vi "laneleftright41.vi"() -> (2 "Coeff right":dbl[](array[numeric]), 3 "Coeff left":dbl[](array[numeric]))   [LabVIEW 2015]
uses:
  G_SEN.vi
  <vilib>/Analysis/1siggen.llb/Ramp Pattern by Delta.vi
  G_LCM.vi
  <vilib>/Analysis/polynomials.llb/1D Polynomial Evaluation (DBL).vi
  G_ALL.vi
  <vilib>/Analysis/NI_AALPro.lvlib
  <vilib>/Analysis/NI_AALBase.lvlib
panel:
  out "y 2":dbl[](array[numeric])
  out "x 2":dbl[](array[numeric])
  out "w 2":dbl[](array[numeric])
  out "lane_right_pt":dbl[][](array[numeric])
  in  "x_gain":dbl=1.0 min=-1.0 max=1.0
  in  "y_gain":dbl=1.0 min=-1.0 max=1.0
  out "map_track 2":dbl[][](array[numeric])
  in  "d_safe":dbl=1.1 format="%#_13g"
  out "map_track":dbl[][](array[numeric])
  out "lane_left_pt":dbl[][](array[numeric])
  out "x_shift":dbl format="%#_13g"
  out "y_shift":dbl format="%#_13g"
  in  "lane_gain":dbl=0.7 min=-1.0 max=1.0
  out "Lane_C_M":dbl[](array[numeric])=[0.8601491478953653, 0.8717844136967624, 0.882947592858927, 0.8936326403234123, 0.9038337699485205, 0.9135454576426009, 0.9227624443554423, 0.9314797389261423, 0.9396926207859084, 0.9473966425143293, 0.9545876322477319, 0.9612616959383189, 0.9674152194628639, 0.9730448705798238, 0.9781476007338057, 0.9827206467064133, 0.9867615321125792, 0.9902680687415704, 0.993238357741943, 0.9956707906498045, 0.9975640502598242, 0.9989171113385246, 0.9997292411794617, 1.0, 0.9997292411794617, 0.9989171113385246, 0.9975640502598242, 0.9956707906498045, 0.993238357741943, 0.9902680687415704, 0.9867615321125792, 0.9827206467064133]
  out "ratio(-1:left1:right)":dbl
  out "NaN/Path/Refnum?":bool
  out "Rleft":dbl
  out "Rright":dbl
  in  "poly":i32=2 min=1 max=5 step=1
  out "Coeff stop":dbl[](array[numeric])
  out "y_end":dbl[](array[numeric])=[0.8601491478953653, 0.8717844136967624, 0.882947592858927, 0.8936326403234123, 0.9038337699485205, 0.9135454576426009, 0.9227624443554423, 0.9314797389261423, 0.9396926207859084, 0.9473966425143293, 0.9545876322477319, 0.9612616959383189, 0.9674152194628639, 0.9730448705798238, 0.9781476007338057, 0.9827206467064133, 0.9867615321125792, 0.9902680687415704, 0.993238357741943, 0.9956707906498045, 0.9975640502598242, 0.9989171113385246, 0.9997292411794617, 1.0, 0.9997292411794617, 0.9989171113385246, 0.9975640502598242, 0.9956707906498045, 0.993238357741943, 0.9902680687415704, 0.9867615321125792, 0.9827206467064133]
  in  "iter":i32=7
  out "Waveform Graph":dbl[](graph)
  out "w":dbl[](array[numeric])
  out "XY Graph 4":cluster{"Y":dbl[], "Y":dbl[]}[](graph)=[{"Y"=array[3210 elements], "Y"=array[3210 elements]}, {"Y"=[-0.0, 0.001154394197769193, 0.004617650635850623, 0.010389990872226917, 0.018471784248973222, 0.02886354801042046, 0.041565947468740205, 0.056579796217107514, 0.0739060563904701, 0.0935458389742223, 0.11550040416098284, 0.13977116175580306, 0.16635967162997645, 0.19526764422393228, 0.2264969410994837, 0.26004957554195585, 0.2959277132125635, 0.3341336728515216, 0.374669927032528, 0.417539102969144, 0.4627439833735707, 0.5102875073687159, 0.560172771454063, 0.6124030305261954, 0.6669816989546717, 0.7239123517142048, 0.7831987255740245, 0.8448447203451934, 0.9088544001870815, 0.975231994973953, 1.0439819017227023, 1.1151086860829622, 1.1886170838907617, 1.2645120027869723, 1.342798523901962, 1.42348190360768, 1.5065675753387922, 1.592061151484188, 1.6799684253507792, 1.770295373200753, 1.8630481563645134, 1.9582331234307588, 2.0558568125157564, 2.1559259536137603, 2.258447471030621], "Y"=[0.0, 0.5, 1.0, 1.5, 2.0, 2.5, 3.0, 3.5, 4.0, 4.5, 5.0, 5.5, 6.0, 6.5, 7.0, 7.5, 8.0, 8.5, 9.0, 9.5, 10.0, 10.5, 11.0, 11.5, 12.0, 12.5, 13.0, 13.5, 14.0, 14.5, 15.0, 15.5, 16.0, 16.5, 17.0, 17.5, 18.0, 18.5, 19.0, 19.5, 20.0, 20.5, 21.0, 21.5, 22.0]}, {"Y"=[0.362252581831572], "Y"=[-0.8199241909738847]}, {"Y"=array[210 elements], "Y"=array[210 elements]}, {"Y"=[-0.925, -0.925, -0.925, -0.6775, -0.6775, -0.925, -0.925, -0.925, -0.925, -0.6775, -0.6775, -0.925, -0.925, -0.925, 0.9025, 0.9025, 0.9025, 0.6775, 0.6775, 0.9025, 0.9025, 0.9025, 0.9025, 0.6775, 0.6775, 0.9025, 0.9025, 0.9025, -0.925], "Y"=[-0.75, -0.224, 0.224, 0.224, -0.224, -0.224, 0.224, 2.415, 2.885, 2.885, 2.415, 2.415, 2.885, 3.5, 3.5, 2.885, 2.415, 2.415, 2.885, 2.885, 2.415, 0.224, -0.224, -0.224, 0.224, 0.224, -0.224, -0.75, -0.75]}, {"Y"=[0.171875, 0.15377271904051304, 0.1346290179491043, 0.11445423440635205, 0.09325870609283447, 0.07105277068912982, 0.04784676587581635, 0.02365102933347224, -0.0015241012573242174, -0.02766828821599482, -0.05477119386196136, -0.08282248051464558, -0.11181181049346922, -0.14172884611785413, -0.17256324970722198, -0.20430468358099463, -0.23694281005859374, -0.27046729145944115, -0.30486779010295867, -0.340133968308568, -0.3762554883956909, -0.41322201268374914, -0.4510232034921646, -0.4896487231403589], "Y"=[0.0, 0.5, 1.0, 1.5, 2.0, 2.5, 3.0, 3.5, 4.0, 4.5, 5.0, 5.5, 6.0, 6.5, 7.0, 7.5, 8.0, 8.5, 9.0, 9.5, 10.0, 10.5, 11.0, 11.5]}, {"Y"=[1.796875, 1.778772719040513, 1.7596290179491043, 1.739454234406352, 1.7182587060928345, 1.6960527706891297, 1.6728467658758164, 1.6486510293334722, 1.6234758987426758, 1.5973317117840051, 1.5702288061380387, 1.5421775194853544, 1.513188189506531, 1.483271153882146, 1.452436750292778, 1.4206953164190055, 1.3880571899414063, 1.354532708540559, 1.3201322098970414, 1.284866031691432, 1.248744511604309, 1.2117779873162509, 1.1739767965078354, 1.135351276859641, 1.0959117660522462, 1.0556686017662287, 1.014632121682167, 0.9728126634806396, 0.9302205648422242, 0.8868661634474992], "Y"=[0.0, 0.5, 1.0, 1.5, 2.0, 2.5, 3.0, 3.5, 4.0, 4.5, 5.0, 5.5, 6.0, 6.5, 7.0, 7.5, 8.0, 8.5, 9.0, 9.5, 10.0, 10.5, 11.0, 11.5, 12.0, 12.5, 13.0, 13.5, 14.0, 14.5]}, {"Y"=[-1.453125, -1.471227280959487, -1.4903709820508957, -1.510545765593648, -1.5317412939071655, -1.5539472293108703, -1.5771532341241836, -1.6013489706665278, -1.6265241012573242, -1.6526682882159949, -1.6797711938619613, -1.7078224805146456, -1.736811810493469, -1.766728846117854, -1.797563249707222, -1.8293046835809945, -1.8619428100585937, -1.895467291459441, -1.9298677901029586], "Y"=[0.0, 0.5, 1.0, 1.5, 2.0, 2.5, 3.0, 3.5, 4.0, 4.5, 5.0, 5.5, 6.0, 6.5, 7.0, 7.5, 8.0, 8.5, 9.0]}, {"Y"=[0.171875, 0.2568230007600336, 0.3384052130063493, 0.44574342526006827, 0.5205081969556753, 0.5917680690742042, 0.659409530134929, 0.7229937549325056, 0.7835496148685115, 0.8405449546633443, 0.9258576868463875], "Y"=[-20.239964538708662, -19.725637940364884, -19.211158961966362, -18.6998967366845, -18.19022720070031, -17.681887266143153, -17.17615515566314, -16.67683575591291, -16.176265245349786, -15.679082775270938, -15.183754484614711]}, {"Y"=[7.134647485270904], "Y"=[38.71960961082238]}, {"Y"=array[980 elements], "Y"=array[980 elements]}, {"Y"=[], "Y"=[]}]
  out "y":dbl[](array[numeric])
  out "x":dbl[](array[numeric])
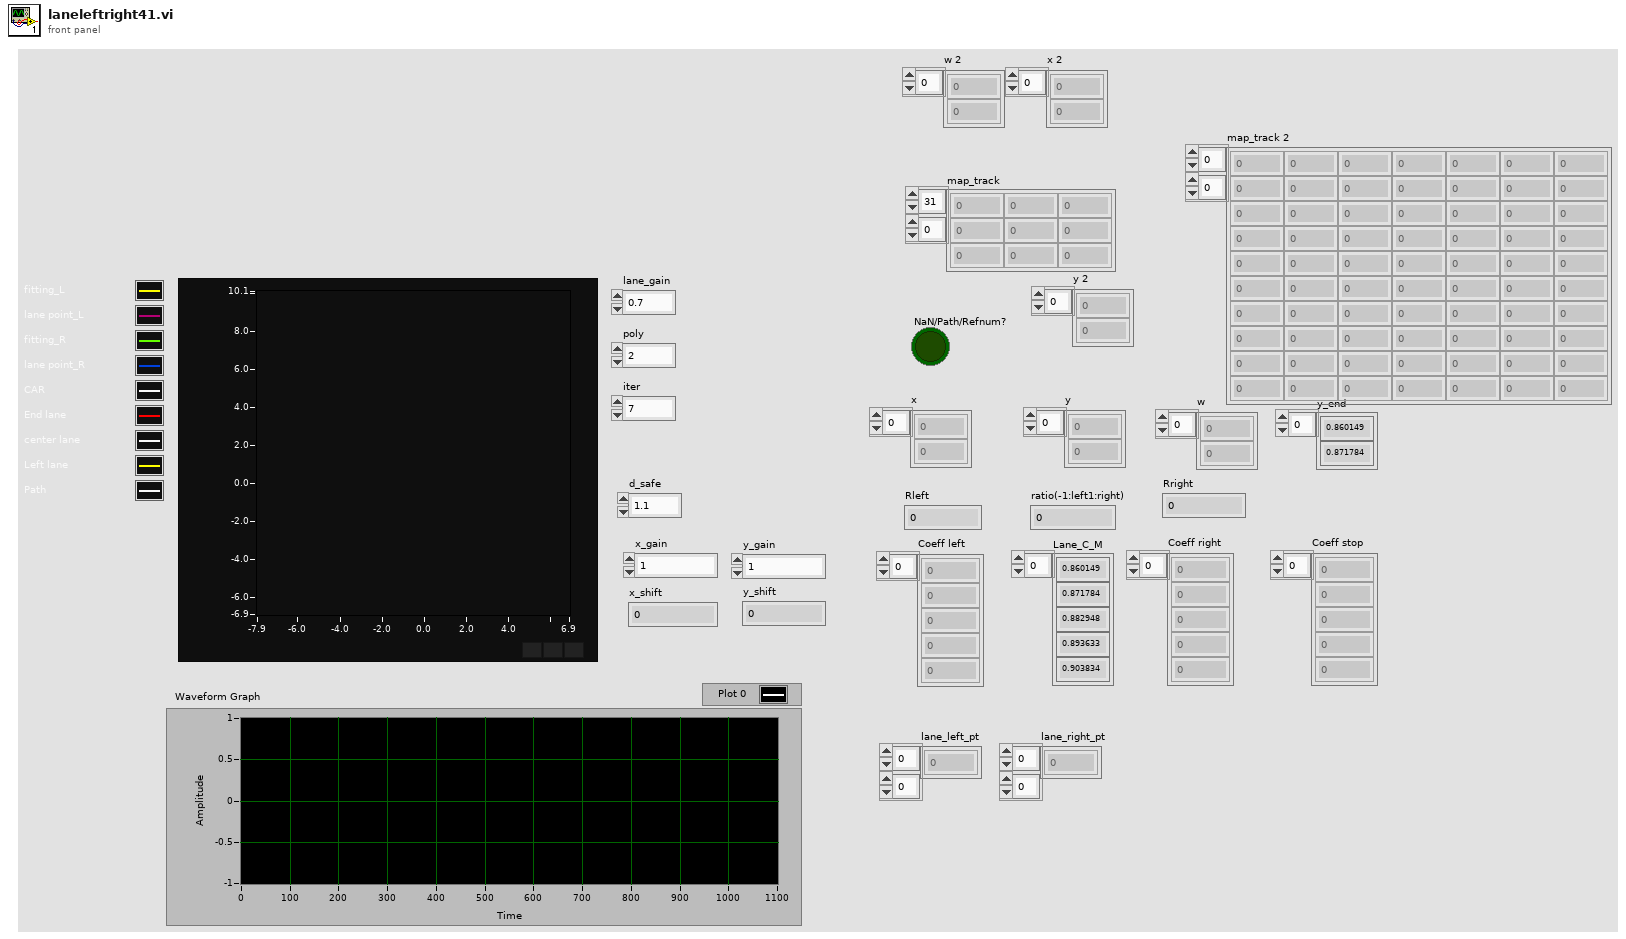
[diagram p1: front panel]
types:
  T1 = cluster{"hash":i64, "sys time":i64, "size":i64, "x":dbl[], "y":dbl[]}
  T2 = cluster{"delta":bool, "Rotational position":dbl, "Rotational position":dbl}[]
  T3 = cluster{"C_Wheel base":dbl, "ratio_steer":dbl, "Overall width":dbl, "af":dbl, "turn radius":dbl, "eval":dbl, "ap":dbl, "an":dbl, "Vmax":dbl, "mu":dbl, "Vlast":dbl}
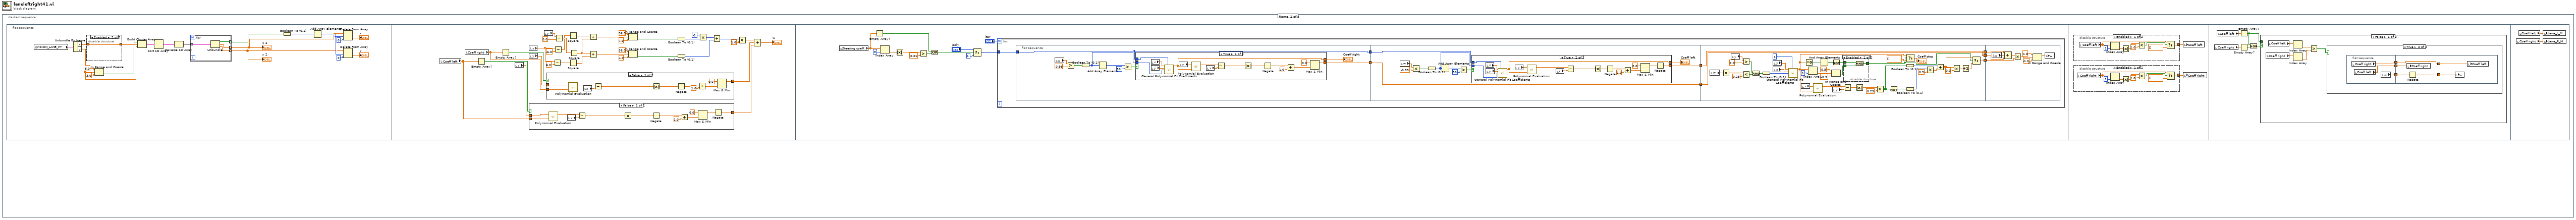
[diagram p0: block diagram]
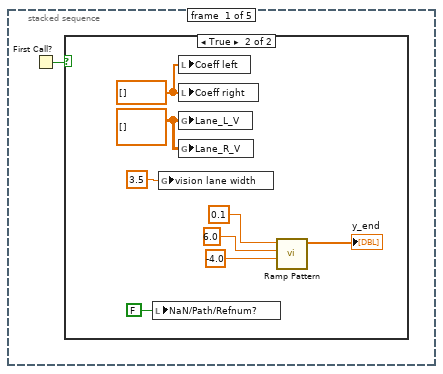
[diagram p2: hidden frame]
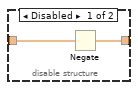
[diagram p4: hidden frame]
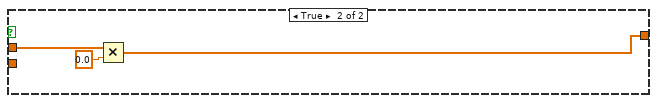
[diagram p5: hidden frame]
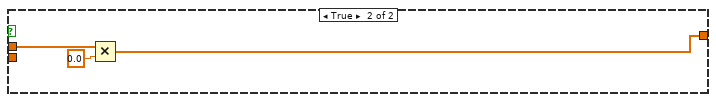
[diagram p6: hidden frame]
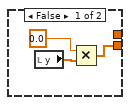
[diagram p7: hidden frame]
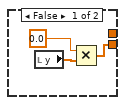
[diagram p8: hidden frame]
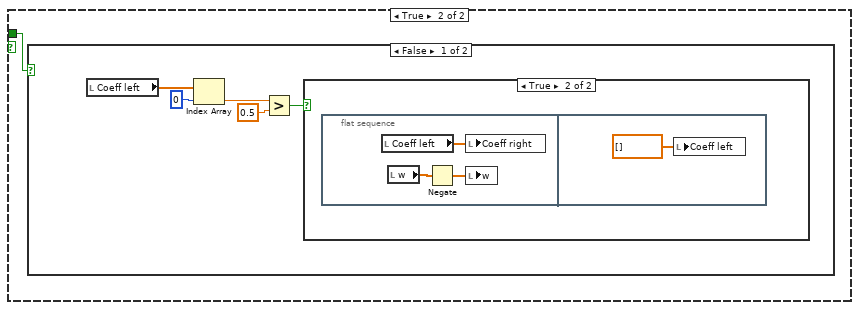
[diagram p13: hidden frame]
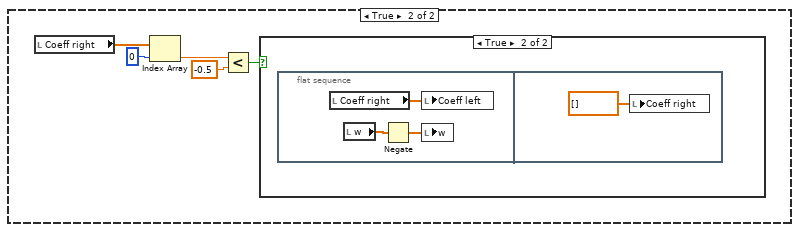
[diagram p15: hidden frame]
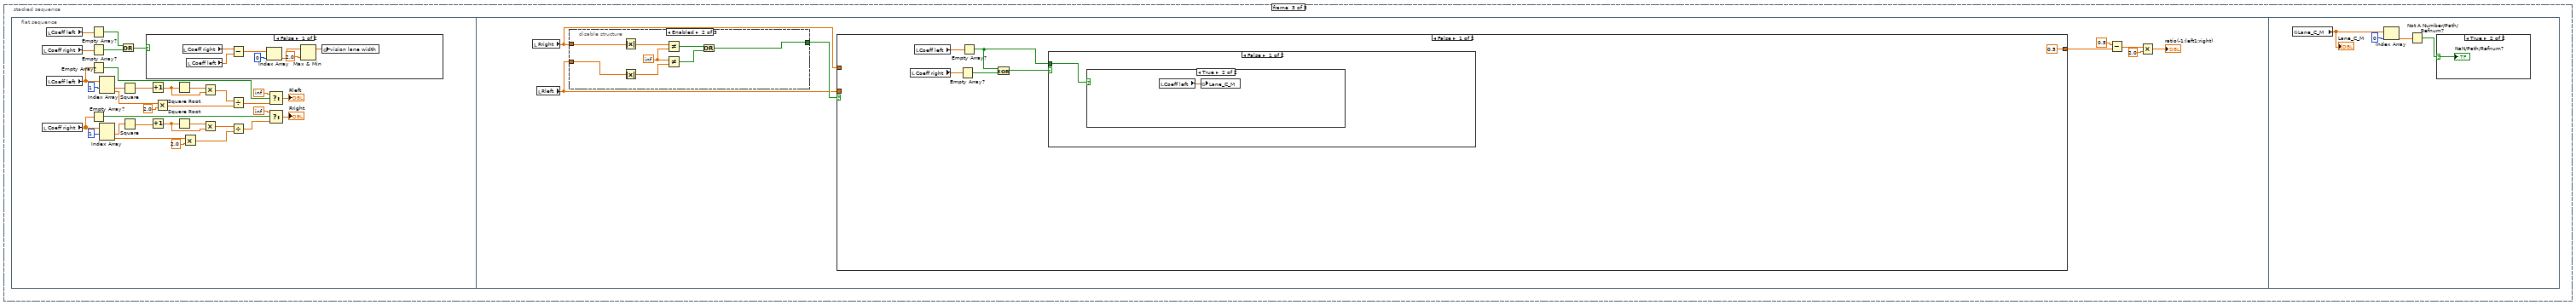
[diagram p17: hidden frame]
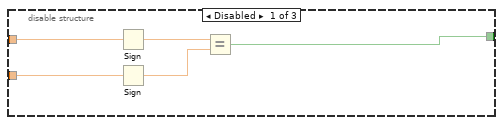
[diagram p19: hidden frame]
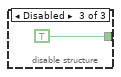
[diagram p20: hidden frame]
diagram:
  n1 = stacked-sequence {
    frame #0 {
      n2 = First Call?() -> (First Call?: T/F=w1:bool)
      n3 = case shown="True" w1 {
        frame False {
        }
        frame True {
          w2 = dbl[] [] ("Coeff left")
          w4 = dbl[][] [] ("Lane_R_V")
          n4 = local write "NaN/Path/Refnum?"(FALSE ("NaN/Path/Refnum?")) -> ()
          n5 = global write "G_SEN.vi" "vision lane width"(3.5 ("vision lane width")) -> ()
          n6 = local write "Coeff left"(w2) -> ()
          n7 = local write "Coeff right"(w2) -> ()
          n8 = global write "G_SEN.vi" "Lane_L_V"(w4) -> ()
          n9 = global write "G_SEN.vi" "Lane_R_V"(w4) -> ()
          n10 = call-poly <vilib>:"Ramp Pattern.vi"("start"=-4.0, "end"=6.0, "delta"=0.1) -> ("Ramp Pattern"=→"y_end":dbl[])  [unwired: 6 in, 2 out]
        }
      }
    }
    frame #1 {
      n11 = flat-sequence {
        frame #0 {
          n12 = global read "G_LCM.vi" "VISION_LANE_PT"() -> (w12:T1)
          n13 = Unbundle By Name(w12) -> ("x"=w27:dbl[], "y"=w21:dbl[])
          n14 = disable-structure shown="Enabled" {
            disable-tunnel: w27 -> [w30 w31]
            disable-tunnel: [w29 w31] -> w28
            frame Disabled {
              n15 = Negate(x=w30) -> (-x=w29:dbl[])
            }
            frame Enabled {
            }
          }
          n16 = In Range and Coerce(upper limit=8.0 ("delta"), x=w21, lower limit=-3.0) -> (In Range?=w19:bool[])  [unwired: 1 out]
          n17 = Build Cluster Array(w19, w28, w21) -> (w17:T2)
          n18 = Sort 1D Array(array=w17) -> (sorted array=w18:T2)
          n19 = Reverse 1D Array(array=w18) -> (reversed array=w14:T2)
          n20 = for {
            tunnel: w14 -> [w35] mode=indexing
            tunnel: [w34] -> w11 mode=indexing
            tunnel: [w33] -> w10 mode=indexing
            tunnel: [w32] -> w22 mode=indexing
            n21 = Unbundle(w35) -> ("delta"=w32:bool, "Rotational position"=w34:dbl, "Rotational position"=w33:dbl)
          }
          "x 2" <- w11
          "y 2" <- w10
          n22 = Boolean To (0,1)(Boolean=w22) -> (0, 1=w15:i16[])
          n23 = Add Array Elements(numeric array=w15) -> (sum=w23:i16)
          n24 = Delete From Array(array=w11, length=w23, index=0) -> (deleted portion=→"x":dbl[])  [unwired: 1 out]
          n25 = Delete From Array(array=w10, length=w23, index=0) -> (deleted portion=→"y":dbl[])  [unwired: 1 out]
        }
        frame #1 {
          n26 = local read "Coeff left"() -> (w67:dbl[])
          n27 = local read "Coeff right"() -> (w66:dbl[])
          n28 = Empty Array?(array=w67) -> (empty?=w68:bool)
          n29 = Empty Array?(array=w66) -> (empty?=w69:bool)
          n30 = local read "y"() -> (w64:dbl[])
          n31 = local read "x"() -> (w36:dbl[])
          n32 = local read "y"() -> (w70:dbl[])
          n33 = case shown="False" w68 {
            tunnel: w64 -> [w90 w98]
            tunnel: w67 -> [w87 _]
            tunnel: [w85 w97] -> w65
            frame False {
              n34 = call-poly <vilib>:"Polynomial Evaluation.vi"("P(x)"=w87, "A"=w90) -> ("P(A)"=w89:dbl[])  [unwired: 1 out]
              n35 = local read "x"() -> (w88:dbl[])
              n36 = Subtract(x=w89, y=w88) -> (x-y=w94:dbl[])
              n37 = Absolute Value(x=w94) -> (abs(x)=w93:dbl[])
              n38 = Negate(x=w93) -> (-x=w92:dbl[])
              n39 = Add(x=w92, y=1.0) -> (x+y=w96:dbl[])
              n40 = Max & Min(x=0.0, y=w96) -> (max(x,y)=w86:dbl[])  [unwired: 1 out]
              n41 = Negate(x=w86) -> (-x=w85:dbl[])
            }
            frame True {
              n42 = Multiply(x=w98, y=0.0) -> (x*y=w97:dbl[])
            }
          }
          n43 = local read "y"() -> (w37:dbl[])
          n44 = case shown="False" w69 {
            tunnel: [w79 w82] -> w62
            tunnel: w66 -> [w78 _]
            tunnel: w70 -> [w71 w83]
            frame False {
              n45 = call-poly <vilib>:"Polynomial Evaluation.vi"("P(x)"=w78, "A"=w71) -> ("P(A)"=w76:dbl[])  [unwired: 1 out]
              n46 = local read "x"() -> (w77:dbl[])
              n47 = Subtract(x=w76, y=w77) -> (x-y=w72:dbl[])
              n48 = Absolute Value(x=w72) -> (abs(x)=w73:dbl[])
              n49 = Negate(x=w73) -> (-x=w74:dbl[])
              n50 = Add(x=w74, y=1.0) -> (x+y=w80:dbl[])
              n51 = Max & Min(x=0.0, y=w80) -> (max(x,y)=w79:dbl[])  [unwired: 1 out]
            }
            frame True {
              n52 = Multiply(x=w83, y=0.0) -> (x*y=w82:dbl[])
            }
          }
          n53 = Subtract(x=w36, y=6.0) -> (x-y=w40:dbl[])
          n54 = Subtract(x=w36, y=-6.0) -> (x-y=w42:dbl[])
          n55 = Subtract(x=w37, y=0.0) -> (x-y=w49:dbl[])
          n56 = Square(x=w42) -> (x^2=w41:dbl[])
          n57 = Square(x=w40) -> (x^2=w50:dbl[])
          n58 = Square(x=w49) -> (x^2=w51:dbl[])
          n59 = Add(x=w41, y=w51) -> (x+y=w57:dbl[])
          n60 = Add(x=w51, y=w50) -> (x+y=w52:dbl[])
          n61 = In Range and Coerce(upper limit=36.0, x=w57, lower limit=4.0) -> (In Range?=w59:bool[])  [unwired: 1 out]
          n62 = In Range and Coerce(upper limit=36.0, x=w52, lower limit=4.0) -> (In Range?=w58:bool[])  [unwired: 1 out]
          n63 = Boolean To (0,1)(Boolean=w59) -> (0, 1=w60:i16[])
          n64 = Boolean To (0,1)(Boolean=w58) -> (0, 1=w61:i16[])
          n65 = Multiply(x=i16 -1, y=w60) -> (x*y=w45:i16[])
          n66 = Add(x=w45, y=w61) -> (x+y=w47:i16[])
          n67 = Multiply(x=w47, y=1.0 ("element")) -> (x*y=w63:dbl[])
          n68 = Compound Arithmetic op=ADD(w63, w62, w65) -> (→"w":dbl[])
        }
        frame #2 {
          n69 = global read "G_ALL.vi" "Steering coeff"() -> (w107:dbl[])
          n70 = Empty Array?(array=w107) -> (empty?=w110:bool)
          n71 = Index Array(array=w107, index=3) -> (element=w105:dbl)
          n72 = Absolute Value(x=w105) -> (abs(x)=w104:dbl)
          n73 = Greater?(x=w104, y=0.01) -> (0:w102:bool)
          n74 = Or(x=w110, y=w102) -> (x .or. y?=w109:bool)
          n75 = Select(t="poly", s=w109, f=1) -> (s? t:f=w100:i32)
          n76 = for {
            N: "iter" -> [_]
            tunnel: w100 -> [w113]
            n77 = flat-sequence {
              tunnel: [w127] -> w119
              tunnel: w113 -> [w120]
              tunnel: [w120] -> w112
              tunnel: [w158] -> w118
              tunnel: w119 -> [w158]
              tunnel: [w155] -> w116
              tunnel: w112 -> [w148]
              tunnel: w118 -> [w220]
              tunnel: [w220] -> w117
              tunnel: w116 -> [w219]
              tunnel: [w219] -> w115
              tunnel: [w190] -> w114
              tunnel: w117 -> [w228]
              tunnel: w115 -> [w224]
              tunnel: w114 -> [w226]
              frame #0 {
                n78 = local read "w"() -> (w129:dbl[])
                n79 = Greater?(x=w129, y=0.99) -> (0:w121:bool[])
                n80 = Boolean To (0,1)(Boolean=w121) -> (0, 1=w122:i16[])
                n81 = Add Array Elements(numeric array=w122) -> (sum=w125:i16)
                n82 = Greater?(x=w125, y=i16 50) -> (0:w123:bool)
                n83 = case shown="True" w123 {
                  tunnel: [w131 w138] -> w127
                  tunnel: [_ w137] -> w126
                  tunnel: w122 -> [_ w134]
                  tunnel: w120 -> [_ w133]
                  frame False {
                    n84 = local read "y"() -> (w132:dbl[])
                    n85 = Multiply(x=0.0, y=w132) -> (x*y=w131:dbl[])
                  }
                  frame True {
                    n86 = local read "x"() -> (w135:dbl[])
                    n87 = local read "y"() -> (w136:dbl[])
                    n88 = call <vilib>:"General Polynomial Fit Coefficients.vi"("Y"=w135, "polynomial order"=w133, "X"=w136, "Weight"=w134) -> ("Polynomial Coefficients"=w137:dbl[])  [unwired: 10 in, 1 out]
                    n89 = local read "y"() -> (w147:dbl[])
                    n90 = call-poly <vilib>:"Polynomial Evaluation.vi"("P(x)"=w137, "A"=w147) -> ("P(A)"=w146:dbl[])  [unwired: 1 out]
                    n91 = local read "x"() -> (w145:dbl[])
                    n92 = Subtract(x=w146, y=w145) -> (x-y=w144:dbl[])
                    n93 = Absolute Value(x=w144) -> (abs(x)=w143:dbl[])
                    n94 = Negate(x=w143) -> (-x=w142:dbl[])
                    n95 = Add(x=w142, y=1.0) -> (x+y=w139:dbl[])
                    n96 = Max & Min(x=0.0, y=w139) -> (max(x,y)=w138:dbl[])  [unwired: 1 out]
                  }
                }
                "Coeff right" <- w126
              }
              frame #1 {
                n97 = local read "w"() -> (w156:dbl[])
                n98 = Less?(x=w156, y=-0.99) -> (x < y?=w151:bool[])
                n99 = Boolean To (0,1)(Boolean=w151) -> (0, 1=w149:i16[])
                n100 = Add Array Elements(numeric array=w149) -> (sum=w152:i16)
                n101 = Greater?(x=w152, y=i16 50) -> (0:w150:bool)
                n102 = case shown="True" w150 {
                  tunnel: [w159 w167] -> w155
                  tunnel: [_ w166] -> w154
                  tunnel: w149 -> [_ w163]
                  tunnel: w148 -> [_ w162]
                  frame False {
                    n103 = local read "y"() -> (w160:dbl[])
                    n104 = Multiply(x=0.0, y=w160) -> (x*y=w159:dbl[])
                  }
                  frame True {
                    n105 = local read "x"() -> (w164:dbl[])
                    n106 = local read "y"() -> (w165:dbl[])
                    n107 = call <vilib>:"General Polynomial Fit Coefficients.vi"("Y"=w164, "polynomial order"=w162, "X"=w165, "Weight"=w163) -> ("Polynomial Coefficients"=w166:dbl[])  [unwired: 10 in, 1 out]
                    n108 = local read "y"() -> (w171:dbl[])
                    n109 = call-poly <vilib>:"Polynomial Evaluation.vi"("P(x)"=w166, "A"=w171) -> ("P(A)"=w172:dbl[])  [unwired: 1 out]
                    n110 = local read "x"() -> (w173:dbl[])
                    n111 = Subtract(x=w172, y=w173) -> (x-y=w174:dbl[])
                    n112 = Absolute Value(x=w174) -> (abs(x)=w175:dbl[])
                    n113 = Negate(x=w175) -> (-x=w169:dbl[])
                    n114 = Add(x=w169, y=1.0) -> (x+y=w176:dbl[])
                    n115 = Max & Min(x=0.0, y=w176) -> (max(x,y)=w170:dbl[])  [unwired: 1 out]
                    n116 = Negate(x=w170) -> (-x=w167:dbl[])
                  }
                }
                "Coeff left" <- w154
              }
              frame #2 {
                n117 = local read "w"() -> (w198:dbl[])
                n118 = Absolute Value(x=w198) -> (abs(x)=w197:dbl[])
                n119 = local read "y"() -> (w202:dbl[])
                n120 = Greater?(x=w202, y=2.0) -> (0:w200:bool[])
                n121 = Less?(x=w197, y=0.25) -> (x < y?=w196:bool[])
                n122 = And(x=w200, y=w196) -> (x .and. y?=w199:bool[])
                n123 = Boolean To (0,1)(Boolean=w199) -> (0, 1=w218:i16[])
                n124 = local read "y"() -> (w212:dbl[])
                n125 = local read "x"() -> (w211:dbl[])
                n126 = call <vilib>:"General Polynomial Fit Coefficients.vi"("Y"=w212, "polynomial order"=1, "X"=w211, "Weight"=w218) -> ("Polynomial Coefficients"=w183:dbl[])  [unwired: 10 in, 1 out]
                n127 = local read "x"() -> (w216:dbl[])
                n128 = Equal To 0?(x=w183) -> (x = 0?=w182:bool[])
                n129 = Index Array(array=w183, index=1) -> (element=w193:dbl)
                n130 = call-poly <vilib>:"Polynomial Evaluation.vi"("P(x)"=w183, "A"=w216) -> ("P(A)"=w215:dbl[])  [unwired: 1 out]
                n131 = And Array Elements(Boolean array=w182) -> (logical AND=w179:bool)
                n132 = In Range and Coerce(upper limit=0.5, x=w193, lower limit=-0.5) -> (In Range?=w181:bool)  [unwired: 1 out]
                n133 = Not(x=w179) -> (.not. x?=w178:bool)
                n134 = local read "y"() -> (w214:dbl[])
                n135 = Subtract(x=w215, y=w214) -> (x-y=w213:dbl[])
                n136 = disable-structure shown="Enabled" {
                  disable-tunnel: w181 -> [w223 _]
                  disable-tunnel: [w222 _] -> w180
                  disable-tunnel: w178 -> [w221 _]
                  frame Enabled {
                    n137 = And(x=w221, y=w223) -> (x .and. y?=w222:bool)
                  }
                  frame Disabled {
                  }
                }
                n138 = Absolute Value(x=w213) -> (abs(x)=w210:dbl[])
                n139 = Greater?(x=w210, y=0.25 ("Numeric 2")) -> (0:w208:bool[])
                n140 = Not(x=w208) -> (.not. x?=w207:bool[])
                n141 = Boolean To (0,1)(Boolean=w208) -> (0, 1=w203:i16[])
                n142 = Boolean To (0,1)(Boolean=w207) -> (0, 1=w206:i16[])
                n143 = Select(t=w183, s=w180, f=dbl[] []) -> (s? t:f=→"Coeff stop":dbl[])
                n144 = Multiply(x=w206, y=0.5) -> (x*y=w204:dbl[])
                n145 = Add(x=w203, y=w204) -> (x+y=w189:dbl[])
                n146 = Multiply(x=w189, y=0.0) -> (x*y=w187:dbl[])
                n147 = Increment(x=w187) -> (x+1=w186:dbl[])
                n148 = Select(t=w189, s=w180, f=w186) -> (s? t:f=w190:dbl[])
              }
              frame #3 {
                n149 = local read "w"() -> (w232:dbl[])
                n150 = Compound Arithmetic op=ADD(w224, w232, w228) -> (w225:dbl[])
                n151 = Multiply(x=w225, y=w226) -> (x*y=w227:dbl[])
                n152 = In Range and Coerce(upper limit=1.0, x=w227, lower limit=-1.0) -> (coerced(x)=w229:dbl[])  [unwired: 1 out]
                n153 = local write "w"(w229) -> ()
              }
            }
          }
        }
        frame #3 {
          n154 = disable-structure shown="Enabled" {
            disable-tunnel: [w236 _] -> w233
            frame Enabled {
              n155 = local read "Coeff left"() -> (w235:dbl[])
              n156 = Index Array(array=w235, index=1) -> (element=w238:dbl)
              n157 = Absolute Value(x=w238) -> (abs(x)=w239:dbl)
              n158 = Less?(x=w239, y=1.0) -> (x < y?=w241:bool)
              n159 = Select(t=w235, s=w241, f=dbl[] []) -> (s? t:f=w236:dbl[])
            }
            frame Disabled {
            }
          }
          n160 = disable-structure shown="Enabled" {
            disable-tunnel: [w245 _] -> w234
            frame Enabled {
              n161 = local read "Coeff right"() -> (w243:dbl[])
              n162 = Index Array(array=w243, index=1) -> (element=w249:dbl)
              n163 = Absolute Value(x=w249) -> (abs(x)=w248:dbl)
              n164 = Less?(x=w248, y=1.0) -> (x < y?=w246:bool)
              n165 = Select(t=w243, s=w246, f=dbl[] []) -> (s? t:f=w245:dbl[])
            }
            frame Disabled {
            }
          }
          n166 = local write "Coeff left"(w233) -> ()
          n167 = local write "Coeff right"(w234) -> ()
        }
        frame #4 {
          n168 = local read "Coeff right"() -> (w252:dbl[])
          n169 = local read "Coeff left"() -> (w251:dbl[])
          n170 = Empty Array?(array=w251) -> (empty?=w255:bool)
          n171 = Empty Array?(array=w252) -> (empty?=w253:bool)
          n172 = Exclusive Or(1:w253, 2:w255) -> (0:w254:bool)
          n173 = case shown="False" w254 {
            tunnel: w255 -> [_ w275]
            frame False {
              n174 = local read "Coeff right"() -> (w259:dbl[])
              n175 = local read "Coeff left"() -> (w260:dbl[])
              n176 = Index Array(array=w260) -> (element=w258:dbl)  [unwired: 1 in]
              n177 = Index Array(array=w259) -> (element=w257:dbl)  [unwired: 1 in]
              n178 = Greater?(x=w258, y=w257) -> (0:w256:bool)
              n179 = case shown="True" w256 {
                frame False {
                }
                frame True {
                  n180 = flat-sequence {
                    tunnel: [w268] -> w264
                    tunnel: [w267] -> w263
                    tunnel: [w266] -> w262
                    tunnel: [w272] -> w265
                    tunnel: w264 -> [w272]
                    tunnel: w263 -> [w271]
                    tunnel: w262 -> [w270]
                    tunnel: [w269] -> w261
                    tunnel: w265 -> [w274]
                    tunnel: w261 -> [w273]
                    frame #0 {
                      n181 = local read "Coeff right"() -> (w268:dbl[])
                      n182 = local read "Coeff left"() -> (w267:dbl[])
                      n183 = local read "w"() -> (w266:dbl[])
                    }
                    frame #1 {
                      n184 = local write "Coeff right"(w271) -> ()
                      n185 = Negate(x=w270) -> (-x=w269:dbl[])
                    }
                    frame #2 {
                      n186 = local write "w"(w273) -> ()
                      n187 = local write "Coeff left"(w274) -> ()
                    }
                  }
                }
              }
            }
            frame True {
              n188 = case shown="False" w275 {
                frame False {
                  n189 = local read "Coeff left"() -> (w280:dbl[])
                  n190 = Index Array(array=w280, index=0) -> (element=w278:dbl)
                  n191 = Greater?(x=w278, y=0.5) -> (0:w276:bool)
                  n192 = case shown="True" w276 {
                    frame False {
                    }
                    frame True {
                      n193 = flat-sequence {
                        frame #0 {
                          n194 = local read "Coeff left"() -> (w283:dbl[])
                          n195 = local read "w"() -> (w282:dbl[])
                          n196 = Negate(x=w282) -> (-x=w281:dbl[])
                          n197 = local write "Coeff right"(w283) -> ()
                          n198 = local write "w"(w281) -> ()
                        }
                        frame #1 {
                          n199 = local write "Coeff left"(dbl[] []) -> ()
                        }
                      }
                    }
                  }
                }
                frame True {
                  n200 = local read "Coeff right"() -> (w289:dbl[])
                  n201 = Index Array(array=w289, index=0) -> (element=w287:dbl)
                  n202 = Less?(x=w287, y=-0.5) -> (x < y?=w285:bool)
                  n203 = case shown="True" w285 {
                    frame False {
                    }
                    frame True {
                      n204 = flat-sequence {
                        frame #0 {
                          n205 = local read "Coeff right"() -> (w292:dbl[])
                          n206 = local read "w"() -> (w291:dbl[])
                          n207 = Negate(x=w291) -> (-x=w290:dbl[])
                          n208 = local write "Coeff left"(w292) -> ()
                          n209 = local write "w"(w290) -> ()
                        }
                        frame #1 {
                          n210 = local write "Coeff right"(dbl[] []) -> ()
                        }
                      }
                    }
                  }
                }
              }
            }
          }
        }
        frame #5 {
          n211 = local read "Coeff right"() -> (w295:dbl[])
          n212 = local read "Coeff left"() -> (w294:dbl[])
          n213 = global write "G_SEN.vi" "Lane_L_M"(w294) -> ()
          n214 = global write "G_SEN.vi" "Lane_R_M"(w295) -> ()
        }
      }
    }
    frame #2 {
      n215 = flat-sequence {
        frame #0 {
          n216 = local read "Coeff right"() -> (w297:dbl[])
          n217 = local read "Coeff right"() -> (w325:dbl[])
          n218 = local read "Coeff left"() -> (w296:dbl[])
          n219 = local read "Coeff left"() -> (w323:dbl[])
          n220 = Empty Array?(array=w296) -> (empty?=w299:bool)
          n221 = Empty Array?(array=w297) -> (empty?=w300:bool)
          n222 = Empty Array?(array=w323) -> (empty?=w317:bool)
          n223 = Empty Array?(array=w325) -> (empty?=w319:bool)
          n224 = Index Array(array=w323, index #1=1 ("index")) -> (element #1=w316:dbl, element #2=w309:dbl)  [unwired: 1 in]
          n225 = Index Array(array=w325, index #1=1 ("index")) -> (element #1=w301:dbl, element #2=w308:dbl)  [unwired: 1 in]
          n226 = Or(x=w299, y=w300) -> (x .or. y?=w298:bool)
          n227 = Square(x=w316) -> (x^2=w315:dbl)
          n228 = Square(x=w301) -> (x^2=w302:dbl)
          n229 = case shown="False" w298 {
            frame False {
              n230 = local read "Coeff right"() -> (w332:dbl[])
              n231 = local read "Coeff left"() -> (w329:dbl[])
              n232 = Subtract(x=w332, y=w329) -> (x-y=w330:dbl[])
              n233 = Index Array(array=w330, index=0) -> (element=w333:dbl)
              n234 = Max & Min(x=w333, y=2.0) -> (max(x,y)=w334:dbl)  [unwired: 1 out]
              n235 = global write "G_SEN.vi" "vision lane width"(w334) -> ()
            }
            frame True {
            }
          }
          n236 = Increment(x=w315) -> (x+1=w313:dbl)
          n237 = Increment(x=w302) -> (x+1=w304:dbl)
          n238 = Multiply(x=w309, y=2.0) -> (x*y=w311:dbl)
          n239 = Square Root(x=w313) -> (sqrt(x)=w314:dbl)
          n240 = Square Root(x=w304) -> (sqrt(x)=w303:dbl)
          n241 = Multiply(x=w308, y=2.0) -> (x*y=w306:dbl)
          n242 = Multiply(x=w314, y=w313) -> (x*y=w312:dbl)
          n243 = Multiply(x=w303, y=w304) -> (x*y=w305:dbl)
          n244 = Divide(x=w312, y=w311) -> (x/y=w318:dbl)
          n245 = Divide(x=w305, y=w306) -> (x/y=w320:dbl)
          n246 = Select(t=inf, s=w317, f=w318) -> (s? t:f=→"Rleft":dbl)
          n247 = Select(t=inf, s=w319, f=w320) -> (s? t:f=→"Rright":dbl)
        }
        frame #1 {
          n248 = local read "Rright"() -> (w336:dbl)
          n249 = local read "Rleft"() -> (w337:dbl)
          n250 = disable-structure shown="Enabled" {
            disable-tunnel: w336 -> [w348 w355 _]
            disable-tunnel: w337 -> [w347 w356 _]
            disable-tunnel: [w344 w351 TRUE] -> w338
            frame Disabled {
              n251 = Sign(1:w348) -> (0:w346:dbl)
              n252 = Sign(1:w347) -> (0:w345:dbl)
              n253 = Equal?(x=w346, y=w345) -> (x = y?=w344:bool)
            }
            frame Enabled {
              w353 = inf
              n254 = Absolute Value(x=w355) -> (abs(x)=w354:dbl)
              n255 = Absolute Value(x=w356) -> (abs(x)=w352:dbl)
              n256 = Not Equal?(x=w354, y=w353) -> (x != y?=w350:bool)
              n257 = Not Equal?(x=w353, y=w352) -> (x != y?=w349:bool)
              n258 = Or(x=w350, y=w349) -> (x .or. y?=w351:bool)
            }
            frame Disabled {
            }
          }
          n259 = case shown="False" w338 {
            tunnel: w336 -> [_ w394]
            tunnel: w337 -> [_ w393]
            tunnel: [0.5 w392] -> w339
            frame False {
              n260 = local read "Coeff right"() -> (w362:dbl[])
              n261 = local read "Coeff left"() -> (w363:dbl[])
              n262 = Empty Array?(array=w362) -> (empty?=w361:bool)
              n263 = Empty Array?(array=w363) -> (empty?=w359:bool)
              n264 = Exclusive Or(1:w361, 2:w359) -> (0:w360:bool)
              n265 = case shown="False" w360 {
                tunnel: w359 -> [w364 w373]
                frame False {
                  n266 = case shown="True" w364 {
                    frame False {
                      w365 = 0.5
                      n267 = local read "Coeff right"() -> (w369:dbl[])
                      n268 = local read "Coeff left"() -> (w371:dbl[])
                      n269 = Decrement(x=w365) -> (x-1=w370:dbl)
                      n270 = Multiply(x=w371, y=w365) -> (x*y=w368:dbl[])
                      n271 = Multiply(x=w370, y=w369) -> (x*y=w367:dbl[])
                      n272 = Subtract(x=w368, y=w367) -> (x-y=w366:dbl[])
                      n273 = global write "G_SEN.vi" "Lane_C_M"(w366) -> ()
                    }
                    frame True {
                      n274 = local read "Coeff left"() -> (w372:dbl[])
                      n275 = global write "G_SEN.vi" "Lane_C_M"(w372) -> ()
                    }
                  }
                }
                frame True {
                  n276 = case shown="False" w373 {
                    frame False {
                      n277 = global read "G_SEN.vi" "vision lane width"() -> (w376:dbl)
                      n278 = local read "Coeff left"() -> (w382:dbl[])
                      n279 = Index Array(array=w382, index=0) -> (element=w380:dbl)
                      n280 = Multiply(x=w376, y=0.5) -> (x*y=w374:dbl)
                      n281 = Add(x=w380, y=w374) -> (x+y=w379:dbl)
                      n282 = Replace Array Subset(array=w382, new element=w379, index=0) -> (w377:dbl[])
                      n283 = global write "G_SEN.vi" "Lane_C_M"(w377) -> ()
                    }
                    frame True {
                      n284 = global read "G_SEN.vi" "vision lane width"() -> (w385:dbl)
                      n285 = local read "Coeff right"() -> (w391:dbl[])
                      n286 = Index Array(array=w391, index=0) -> (element=w389:dbl)
                      n287 = Multiply(x=w385, y=0.5) -> (x*y=w383:dbl)
                      n288 = Subtract(x=w389, y=w383) -> (x-y=w388:dbl)
                      n289 = Replace Array Subset(array=w391, new element=w388, index=0) -> (w386:dbl[])
                      n290 = global write "G_SEN.vi" "Lane_C_M"(w386) -> ()
                    }
                  }
                }
              }
            }
            frame True {
              n291 = disable-structure shown="Enabled" {
                disable-tunnel: w394 -> [w403 w627]
                disable-tunnel: w393 -> [w402 w626]
                disable-tunnel: [_ w554] -> w392
                frame Disabled {
                  n292 = Absolute Value(x=w403) -> (abs(x)=w425:dbl)
                  n293 = Absolute Value(x=w402) -> (abs(x)=w424:dbl)
                  n294 = global read "G_ALL.vi" "CARSPEC"() -> (w420:T3)
                  n295 = global read "G_ALL.vi" "CARSPEC"() -> (w441:T3)
                  n296 = Build Array(w425, w424) -> (w423:dbl[])
                  n297 = Unbundle By Name(w420) -> ("af"=w419:dbl, "Overall width"=w409:dbl)
                  n298 = Unbundle By Name(w441) -> ("Overall width"=w430:dbl, "af"=w438:dbl, "Overall width"=w426:dbl)
                  n299 = Array Max & Min(array=w423) -> (min value=w416:dbl, min index (indices)=w422:i32)  [unwired: 2 out]
                  n300 = Add(x=w416, y=w430) -> (x+y=w440:dbl)
                  n301 = Square(x=w416) -> (x^2=w407:dbl)
                  n302 = Square(x=w419) -> (x^2=w406:dbl)
                  n303 = Multiply(x=w409, y=0.5) -> (x*y=w408:dbl)
                  n304 = Square(x=w440) -> (x^2=w439:dbl)
                  n305 = Square(x=w438) -> (x^2=w431:dbl)
                  n306 = Subtract(x=w407, y=w406) -> (x-y=w401:dbl)
                  n307 = Multiply(x=w426, y=0.5) -> (x*y=w427:dbl)
                  n308 = Add(x=w439, y=w431) -> (x+y=w437:dbl)
                  n309 = Square Root(x=w401) -> (sqrt(x)=w418:dbl)
                  n310 = global read "G_SEN.vi" "vision lane width"() -> (w412:dbl)
                  n311 = global read "G_SEN.vi" "vision lane width"() -> (w436:dbl)
                  n312 = Subtract(x=w418, y=w409) -> (x-y=w417:dbl)
                  n313 = Square Root(x=w437) -> (sqrt(x)=w435:dbl)
                  n314 = Subtract(x=w416, y=w417) -> (x-y=w411:dbl)
                  n315 = Subtract(x=w435, y=w416) -> (x-y=w434:dbl)
                  n316 = Subtract(x=w412, y=w411) -> (x-y=w413:dbl)
                  n317 = Subtract(x=w436, y=w434) -> (x-y=w433:dbl)
                  n318 = global read "G_SEN.vi" "vision lane width"() -> (w397:dbl)
                  n319 = global read "G_SEN.vi" "vision lane width"() -> (w404:dbl)
                  n320 = Multiply(x=w413, y=0.5) -> (x*y=w415:dbl)
                  n321 = Multiply(x=w433, y=0.5) -> (x*y=w428:dbl)
                  n322 = Compound Arithmetic op=ADD(w415, w408) -> (w405:dbl)
                  n323 = Compound Arithmetic op=ADD(w428, w427) -> (w421:dbl)
                  n324 = Subtract(x=w404, y=w405) -> (x-y=w399:dbl)
                  n325 = Less Than 0?(x=w401) -> (x < 0?=w400:bool)
                  n326 = Multiply(x=0.5 ("y"), y=w397) -> (x*y=w396:dbl)
                  n327 = Select(t=w396, s=w400, f=w399) -> (s? t:f=w398:dbl)
                  n328 = case shown="1" w422 {
                    tunnel: w421 -> [w443 w491]
                    tunnel: w398 -> [w442 w489]
                    frame 0, Default {
                      n329 = local read "Rright"() -> (w445:dbl)
                      n330 = Greater Than 0?(x=w445) -> (x > 0?=w444:bool)
                      n331 = case shown="True" w444 {
                        tunnel: w443 -> [_ w466]
                        tunnel: w442 -> [w448 w465]
                        frame False {
                          n332 = local read "Coeff left"() -> (w447:dbl[])
                          n333 = Empty Array?(array=w447) -> (empty?=w446:bool)
                          n334 = case shown="False" w446 {
                            tunnel: w448 -> [w449 w458]
                            frame False {
                              n335 = global read "G_SEN.vi" "vision lane width"() -> (w457:dbl)
                              n336 = Divide(x=w449, y=w457) -> (x/y=w455:dbl)
                              n337 = local read "Coeff right"() -> (w453:dbl[])
                              n338 = local read "Coeff left"() -> (w456:dbl[])
                              n339 = Decrement(x=w455) -> (x-1=w454:dbl)
                              n340 = Multiply(x=w456, y=w455) -> (x*y=w452:dbl[])
                              n341 = Multiply(x=w454, y=w453) -> (x*y=w451:dbl[])
                              n342 = Subtract(x=w452, y=w451) -> (x-y=w450:dbl[])
                              n343 = global write "G_SEN.vi" "Lane_C_M"(w450) -> ()
                            }
                            frame True {
                              n344 = local read "Coeff right"() -> (w464:dbl[])
                              n345 = Index Array(array=w464, index=0) -> (element=w462:dbl)
                              n346 = Subtract(x=w462, y=w458) -> (x-y=w461:dbl)
                              n347 = Replace Array Subset(array=w464, new element=w461, index=0) -> (w459:dbl[])
                              n348 = global write "G_SEN.vi" "Lane_C_M"(w459) -> ()
                            }
                          }
                        }
                        frame True {
                          n349 = local read "Coeff left"() -> (w468:dbl[])
                          n350 = Empty Array?(array=w468) -> (empty?=w467:bool)
                          n351 = case shown="False" w467 {
                            tunnel: w466 -> [w472 w482]
                            tunnel: w465 -> [w473 _]
                            frame False {
                              n352 = Add(x=w473, y=w472) -> (x+y=w471:dbl)
                              n353 = global read "G_SEN.vi" "vision lane width"() -> (w481:dbl)
                              n354 = Multiply(x=w471, y=0.5) -> (x*y=w469:dbl)
                              n355 = Divide(x=w469, y=w481) -> (x/y=w479:dbl)
                              n356 = local read "Coeff right"() -> (w477:dbl[])
                              n357 = local read "Coeff left"() -> (w480:dbl[])
                              n358 = Decrement(x=w479) -> (x-1=w478:dbl)
                              n359 = Multiply(x=w480, y=w479) -> (x*y=w476:dbl[])
                              n360 = Multiply(x=w478, y=w477) -> (x*y=w475:dbl[])
                              n361 = Subtract(x=w476, y=w475) -> (x-y=w474:dbl[])
                              n362 = global write "G_SEN.vi" "Lane_C_M"(w474) -> ()
                            }
                            frame True {
                              n363 = local read "Coeff right"() -> (w488:dbl[])
                              n364 = Index Array(array=w488, index=0) -> (element=w486:dbl)
                              n365 = Subtract(x=w486, y=w482) -> (x-y=w485:dbl)
                              n366 = Replace Array Subset(array=w488, new element=w485, index=0) -> (w483:dbl[])
                              n367 = global write "G_SEN.vi" "Lane_C_M"(w483) -> ()
                            }
                          }
                        }
                      }
                    }
                    frame 1 {
                      n368 = local read "Rleft"() -> (w492:dbl)
                      n369 = Less Than 0?(x=w492) -> (x < 0?=w490:bool)
                      n370 = case shown="True" w490 {
                        tunnel: w491 -> [_ w513]
                        tunnel: w489 -> [w495 w512]
                        frame False {
                          n371 = local read "Coeff right"() -> (w494:dbl[])
                          n372 = Empty Array?(array=w494) -> (empty?=w493:bool)
                          n373 = case shown="False" w493 {
                            tunnel: w495 -> [w496 w505]
                            frame False {
                              n374 = global read "G_SEN.vi" "vision lane width"() -> (w504:dbl)
                              n375 = Divide(x=w496, y=w504) -> (x/y=w502:dbl)
                              n376 = local read "Coeff right"() -> (w503:dbl[])
                              n377 = local read "Coeff left"() -> (w500:dbl[])
                              n378 = Decrement(x=w502) -> (x-1=w501:dbl)
                              n379 = Multiply(x=w503, y=w502) -> (x*y=w499:dbl[])
                              n380 = Multiply(x=w501, y=w500) -> (x*y=w498:dbl[])
                              n381 = Subtract(x=w499, y=w498) -> (x-y=w497:dbl[])
                              n382 = global write "G_SEN.vi" "Lane_C_M"(w497) -> ()
                            }
                            frame True {
                              n383 = local read "Coeff left"() -> (w511:dbl[])
                              n384 = Index Array(array=w511, index=0) -> (element=w509:dbl)
                              n385 = Add(x=w509, y=w505) -> (x+y=w508:dbl)
                              n386 = Replace Array Subset(array=w511, new element=w508, index=0) -> (w506:dbl[])
                              n387 = global write "G_SEN.vi" "Lane_C_M"(w506) -> ()
                            }
                          }
                        }
                        frame True {
                          n388 = local read "Coeff right"() -> (w515:dbl[])
                          n389 = Empty Array?(array=w515) -> (empty?=w514:bool)
                          n390 = case shown="False" w514 {
                            tunnel: w513 -> [w517 w529]
                            tunnel: w512 -> [w518 _]
                            frame False {
                              n391 = Add(x=w518, y=w517) -> (x+y=w520:dbl)
                              n392 = global read "G_SEN.vi" "vision lane width"() -> (w528:dbl)
                              n393 = Multiply(x=w520, y=0.5) -> (x*y=w516:dbl)
                              n394 = Divide(x=w516, y=w528) -> (x/y=w526:dbl)
                              n395 = local read "Coeff right"() -> (w527:dbl[])
                              n396 = local read "Coeff left"() -> (w524:dbl[])
                              n397 = Decrement(x=w526) -> (x-1=w525:dbl)
                              n398 = Multiply(x=w527, y=w526) -> (x*y=w523:dbl[])
                              n399 = Multiply(x=w525, y=w524) -> (x*y=w522:dbl[])
                              n400 = Subtract(x=w523, y=w522) -> (x-y=w521:dbl[])
                              n401 = global write "G_SEN.vi" "Lane_C_M"(w521) -> ()
                            }
                            frame True {
                              n402 = local read "Coeff left"() -> (w535:dbl[])
                              n403 = Index Array(array=w535, index=0) -> (element=w533:dbl)
                              n404 = Add(x=w533, y=w529) -> (x+y=w532:dbl)
                              n405 = Replace Array Subset(array=w535, new element=w532, index=0) -> (w530:dbl[])
                              n406 = global write "G_SEN.vi" "Lane_C_M"(w530) -> ()
                            }
                          }
                        }
                      }
                    }
                  }
                }
                frame Enabled {
                  n407 = Build Array(w627, w626) -> (w601:dbl[])
                  n408 = global read "G_ALL.vi" "CARSPEC"() -> (w624:T3)
                  n409 = Absolute Value(x=w601) -> (abs(x)=w625:dbl[])
                  n410 = Unbundle By Name(w624) -> ("Overall width"=w623:dbl, "af"=w621:dbl, "Overall width"=w549:dbl)
                  n411 = Array Max & Min(array=w625) -> (max value=w603:dbl, min value=w559:dbl, min index (indices)=w600:i32)  [unwired: 1 out]
                  n412 = global read "G_ALL.vi" "CARSPEC"() -> (w612:T3)
                  n413 = Add(x=w559, y=w623) -> (x+y=w622:dbl)
                  n414 = Index Array(array=w601, index=w600) -> (element=w599:dbl)
                  n415 = Square(x=w621) -> (x^2=w619:dbl)
                  n416 = Not Equal?(x=inf, y=w603) -> (x != y?=w598:bool)
                  n417 = Unbundle By Name(w612) -> ("Overall width"=w543:dbl, "af"=w611:dbl)
                  n418 = Select(t=w603, s=w598, f=w559) -> (s? t:f=w602:dbl)
                  n419 = Square(x=w622) -> (x^2=w620:dbl)
                  n420 = Multiply(x=w549, y=0.5) -> (x*y=w548:dbl)
                  n421 = Add(x=w620, y=w619) -> (x+y=w618:dbl)
                  n422 = Square(x=w602) -> (x^2=w609:dbl)
                  n423 = Square(x=w611) -> (x^2=w610:dbl)
                  n424 = global read "G_SEN.vi" "vision lane width"() -> (w615:dbl)
                  n425 = Subtract(x=w609, y=w610) -> (x-y=w560:dbl)
                  n426 = Square Root(x=w618) -> (sqrt(x)=w617:dbl)
                  n427 = Add(x=w548, y=0.1) -> (x+y=w545:dbl)
                  n428 = Subtract(x=w559, y=w617) -> (x-y=w616:dbl)
                  n429 = Max & Min(x=w560, y=w559) -> (max(x,y)=w558:dbl)  [unwired: 1 out]
                  n430 = global read "G_SEN.vi" "vision lane width"() -> (w607:dbl)
                  n431 = Compound Arithmetic op=ADD(w616, w549, w615) -> (w614:dbl)
                  n432 = Square Root(x=w558) -> (sqrt(x)=w608:dbl)
                  n433 = Multiply(x=0.5, y=w543) -> (x*y=w540:dbl)
                  n434 = Subtract(x=w602, y=w608) -> (x-y=w541:dbl)
                  n435 = Multiply(x=w614, y=0.5) -> (x*y=w546:dbl)
                  n436 = Max & Min(x=w546, y=w545) -> (max(x,y)=w544:dbl)  [unwired: 1 out]
                  n437 = Compound Arithmetic op=ADD(w541, w607) -> (w605:dbl)
                  n438 = Compound Arithmetic op=ADD(0.1 ("value"), w540, w541) -> (w537:dbl)
                  n439 = Multiply(x=w605, y=0.5) -> (x*y=w538:dbl)
                  n440 = Max & Min(x=w537, y=w538) -> (max(x,y)=w536:dbl)  [unwired: 1 out]
                  n441 = case shown="True" w598 {
                    tunnel: w600 -> [w632 w650]
                    tunnel: w599 -> [w631 _]
                    tunnel: w544 -> [w630 w653]
                    tunnel: [w629 w645] -> w597
                    tunnel: w536 -> [w628 w655]
                    frame False {
                      n442 = case shown="1" w632 {
                        tunnel: w631 -> [w637 w644]
                        tunnel: w630 -> [w634 w642]
                        tunnel: [w633 w638] -> w629
                        tunnel: w628 -> [w635 w641]
                        frame 0, Default {
                          n443 = Less Than 0?(x=w637) -> (x < 0?=w636:bool)
                          n444 = Select(t=w635, s=w636, f=w634) -> (s? t:f=w633:dbl)
                        }
                        frame 1 {
                          n445 = Greater Than 0?(x=w644) -> (x > 0?=w643:bool)
                          n446 = global read "G_SEN.vi" "vision lane width"() -> (w640:dbl)
                          n447 = Select(t=w641, s=w643, f=w642) -> (s? t:f=w639:dbl)
                          n448 = Subtract(x=w640, y=w639) -> (x-y=w638:dbl)
                        }
                      }
                    }
                    frame True {
                      n449 = Equal To 0?(x=w650) -> (x = 0?=w649:bool)
                      n450 = global read "G_SEN.vi" "vision lane width"() -> (w656:dbl)
                      n451 = Subtract(x=w656, y=w655) -> (x-y=w654:dbl)
                      n452 = global read "G_SEN.vi" "vision lane width"() -> (w648:dbl)
                      n453 = Add(x=w654, y=w653) -> (x+y=w651:dbl)
                      n454 = Multiply(x=w651, y=0.5) -> (x*y=w647:dbl)
                      n455 = Subtract(x=w648, y=w647) -> (x-y=w646:dbl)
                      n456 = Select(t=w647, s=w649, f=w646) -> (s? t:f=w645:dbl)
                    }
                  }
                  n457 = global read "G_SEN.vi" "vision lane width"() -> (w596:dbl)
                  n458 = local read "Coeff right"() -> (w582:dbl[])
                  n459 = local read "Coeff left"() -> (w569:dbl[])
                  n460 = global read "G_SEN.vi" "vision lane width"() -> (w580:dbl)
                  n461 = global read "G_SEN.vi" "vision lane width"() -> (w571:dbl)
                  n462 = Divide(x=w597, y=w596) -> (x/y=w556:dbl)
                  n463 = local read "poly"() -> (w587:i32)
                  n464 = local read "poly"() -> (w565:i32)
                  n465 = Increment(x=w587) -> (x+1=w586:i32)
                  n466 = Increment(x=w565) -> (x+1=w566:i32)
                  n467 = Index Array(array=w582, index #1=0 ("index")) -> (element #1=w581:dbl, element #2=w562:dbl)  [unwired: 1 in]
                  n468 = Index Array(array=w569, index #1=0 ("index")) -> (element #1=w570:dbl, element #2=w561:dbl)  [unwired: 1 in]
                  n469 = Subtract(x=0.5, y=w556) -> (x-y=w553:dbl)
                  n470 = local read "Coeff right"() -> (w575:dbl[])
                  n471 = Subtract(x=w581, y=w580) -> (x-y=w579:dbl)
                  n472 = Add(x=w570, y=w571) -> (x+y=w572:dbl)
                  n473 = Initialize Array(0.0 ("element"), w586) -> (w585:dbl[])
                  n474 = Initialize Array(0.0 ("element"), w566) -> (w567:dbl[])
                  n475 = local read "Coeff left"() -> (w590:dbl[])
                  n476 = Multiply(x=w553, y="lane_gain") -> (x*y=w552:dbl)
                  n477 = Empty Array?(array=w575) -> (empty?=w577:bool)
                  n478 = Empty Array?(array=w590) -> (empty?=w591:bool)
                  n479 = Replace Array Subset(array=w585, new element #1=w579, index #1=0 ("index"), new element #2=w562) -> (w584:dbl[])  [unwired: 1 in]
                  n480 = Replace Array Subset(array=w567, new element #1=w572, index #1=0 ("index"), new element #2=w561) -> (w563:dbl[])  [unwired: 1 in]
                  n481 = Not(x=w577) -> (.not. x?=w576:bool)
                  n482 = Subtract(x=0.5 ("y"), y=w552) -> (x-y=w554:dbl)
                  n483 = Select(t=w584, s=w591, f=w590) -> (s? t:f=w589:dbl[])
                  n484 = Select(t=w575, s=w576, f=w563) -> (s? t:f=w574:dbl[])
                  n485 = Decrement(x=w554) -> (x-1=w595:dbl)
                  n486 = Multiply(x=w589, y=w554) -> (x*y=w593:dbl[])
                  n487 = Multiply(x=w595, y=w574) -> (x*y=w594:dbl[])
                  n488 = Subtract(x=w593, y=w594) -> (x-y=w592:dbl[])
                  n489 = global write "G_SEN.vi" "Lane_C_M"(w592) -> ()
                }
              }
            }
          }
          n490 = Subtract(x=0.5, y=w339) -> (x-y=w341:dbl)
          n491 = Multiply(x=w341, y=2.0) -> (x*y=→"ratio(-1:left1:right)":dbl)
        }
        frame #2 {
          n492 = global read "G_SEN.vi" "Lane_C_M"() -> (w657:dbl[])
          "Lane_C_M" <- w657
          n493 = Index Array(array=w657, index=0) -> (element=w659:dbl)
          n494 = Not A Number/Path/Refnum?(number/path/refnum=w659) -> (NaN/Path/Refnum?=w660:bool)
          n495 = case shown="True" w660 {
            selector: w660 -> [_ w661]
            frame False {
            }
            frame True {
              "NaN/Path/Refnum?" <- w661
            }
          }
        }
      }
    }
    frame #3 {
      n496 = global read "G_ALL.vi" "map_track 2"() -> (w664:dbl[][])
      n497 = Empty Array?(array=w664) -> (empty?=w662:bool)
      n498 = case shown="False" w662 {
        tunnel: [w670 _] -> w665
        tunnel: [w669 _] -> w666
        tunnel: [w668 _] -> w663
        tunnel: w664 -> [w667 _]
        frame False {
          n499 = flat-sequence {
            tunnel: w667 -> [w671]
            tunnel: [w787] -> w670
            tunnel: [w786] -> w669
            tunnel: [w785] -> w668
            frame #0 {
              n500 = global read "G_ALL.vi" "dist"() -> (w676:dbl[])
              n501 = Threshold 1D Array(2:-4.0 ("threshold y"), 3:w676) -> (0:w674:dbl)  [unwired: 1 in]
              n502 = Round Toward +Infinity(x=w674) -> (ceil(x): smallest int >= x=w672:dbl)
              n503 = Array Subset(array=w671, index (row)=w672) -> (→"map_track":dbl[][])  [unwired: 3 in]
            }
            frame #1 {
              n504 = local read "d_safe"() -> (w683:dbl)
              n505 = local read "y 2"() -> (w680:dbl[])
              n506 = local read "map_track"() -> (w677:dbl[][])
              n507 = Array Size(array=w680) -> (size(s)=w679:i32)
              n508 = local read "x 2"() -> (w684:dbl[])
              n509 = Subtract(x=w683, y=0.2) -> (x-y=w682:dbl)
              n510 = for {
                N: w679 -> [_]
                tunnel: w680 -> [w691] mode=indexing
                tunnel: w684 -> [w692] mode=indexing
                tunnel: w677 -> [w697]
                tunnel: w682 -> [w693]
                tunnel: [w689] -> w685 mode=indexing
                tunnel: [w686] -> w678 mode=indexing
                i -> [w687]
                n511 = Build Array(w692, w691) -> (w690:dbl[])
                n512 = Index Array(array=w697, index (col) #1=0 ("disabled index (col)")) -> (element #1=w705:dbl[], element #2=w704:dbl[])  [unwired: 3 in]
                n513 = Subtract(x=w692, y=w705) -> (x-y=w702:dbl[])
                n514 = Subtract(x=w704, y=w691) -> (x-y=w703:dbl[])
                n515 = Square(x=w702) -> (x^2=w701:dbl[])
                n516 = Square(x=w703) -> (x^2=w700:dbl[])
                n517 = Add(x=w701, y=w700) -> (x+y=w699:dbl[])
                n518 = Square Root(x=w699) -> (sqrt(x)=w698:dbl[])
                n519 = Array Max & Min(array=w698) -> (min value=w694:dbl, min index (indices)=w696:i32)  [unwired: 2 out]
                n520 = Less Or Equal?(x=w693, y=w694) -> (x <= y?=w695:bool)
                n521 = case shown="True" w695 {
                  tunnel: w697 -> [_ w728]
                  tunnel: w696 -> [_ w727]
                  tunnel: w690 -> [_ w721]
                  tunnel: [_ w709] -> w689
                  frame False {
                  }
                  frame True {
                    n522 = Decrement(x=w727) -> (x-1=w726:i32)
                    n523 = Max & Min(x=w726, y=0) -> (max(x,y)=w725:i32)  [unwired: 1 out]
                    n524 = Index Array(array=w728, index (row) #1=w725) -> (element #1=w722:dbl[], element #2=w723:dbl[])  [unwired: 3 in]
                    n525 = Subtract(x=w721, y=w722) -> (x-y=w718:dbl[])
                    n526 = Subtract(x=w723, y=w722) -> (x-y=w720:dbl[])
                    n527 = Index Array(array=w718, index #1=0 ("index"), index #2=1 ("index")) -> (element #1=w712:dbl, element #2=w714:dbl)
                    n528 = Index Array(array=w720, index #1=0 ("index"), index #2=1 ("index")) -> (element #1=w713:dbl, element #2=w711:dbl)
                    n529 = Multiply(x=w712, y=w711) -> (x*y=w708:dbl)
                    n530 = Multiply(x=w714, y=w713) -> (x*y=w707:dbl)
                    n531 = Subtract(x=w708, y=w707) -> (x-y=w710:dbl)
                    n532 = Sign(1:w710) -> (0:w709:dbl)
                  }
                }
                n533 = local read "w"() -> (w688:dbl[])
                n534 = Index Array(array=w688, index=w687) -> (element=w686:dbl)
              }
              "w 2" <- w685
              n535 = local write "w"(w678) -> ()
            }
            frame #2 {
              n536 = local read "w 2"() -> (w746:dbl[])
              n537 = local read "w 2"() -> (w747:dbl[])
              n538 = local read "w"() -> (w749:dbl[])
              n539 = local read "w"() -> (w739:dbl[])
              n540 = local read "w"() -> (w752:dbl[])
              n541 = local read "w"() -> (w736:dbl[])
              n542 = Greater Or Equal?(x=w746, y=1.0) -> (x >= y?=w741:bool[])
              n543 = Greater Or Equal?(x=w749, y=1.0) -> (x >= y?=w743:bool[])
              n544 = Less Or Equal?(x=w739, y=-1.0) -> (x <= y?=w738:bool[])
              n545 = Less Or Equal?(x=w752, y=-1.0) -> (x <= y?=w744:bool[])
              n546 = Greater Or Equal?(x=w736, y=1.0) -> (x >= y?=w734:bool[])
              n547 = Less Or Equal?(x=w747, y=-1.0) -> (x <= y?=w742:bool[])
              n548 = Or(x=w743, y=w741) -> (x .or. y?=w731:bool[])
              n549 = Or(x=w744, y=w742) -> (x .or. y?=w732:bool[])
              n550 = Not(x=w738) -> (.not. x?=w737:bool[])
              n551 = Not(x=w734) -> (.not. x?=w733:bool[])
              n552 = And(x=w731, y=w737) -> (x .and. y?=w729:bool[])
              n553 = And(x=w732, y=w733) -> (x .and. y?=w730:bool[])
              n554 = local read "x 2"() -> (w753:dbl[])
              n555 = local read "y 2"() -> (w754:dbl[])
              n556 = local read "x 2"() -> (w776:dbl[])
              n557 = local read "y 2"() -> (w775:dbl[])
              n558 = Boolean To (0,1)(Boolean=w729) -> (0, 1=w759:i16[])
              n559 = Boolean To (0,1)(Boolean=w730) -> (0, 1=w770:i16[])
              n560 = Build Cluster Array(w729, w753, w754) -> (w755:cluster{bool, dbl, dbl}[])
              n561 = Build Cluster Array(w730, w776, w775) -> (w774:cluster{bool, dbl, dbl}[])
              n562 = To Long Integer(number=w759) -> (32bit integer=w760:i32[])
              n563 = To Long Integer(number=w770) -> (32bit integer=w769:i32[])
              n564 = Add Array Elements(numeric array=w760) -> (sum=w758:i32)
              n565 = Add Array Elements(numeric array=w769) -> (sum=w771:i32)
              n566 = Sort 1D Array(array=w755) -> (sorted array=w756:cluster{bool, dbl, dbl}[])
              n567 = Sort 1D Array(array=w774) -> (sorted array=w773:cluster{bool, dbl, dbl}[])
              n568 = Reverse 1D Array(array=w756) -> (reversed array=w757:cluster{bool, dbl, dbl}[])
              n569 = Reverse 1D Array(array=w773) -> (reversed array=w772:cluster{bool, dbl, dbl}[])
              n570 = for {
                N: w758 -> [_]
                tunnel: w757 -> [w780] mode=indexing
                tunnel: [w779] -> w762 mode=indexing
                tunnel: [w778] -> w761 mode=indexing
                tunnel: [w777] -> _
                i -> [w777]
                n571 = Unbundle(w780) -> (w779:dbl, w778:dbl)  [unwired: 1 out]
              }
              n572 = for {
                N: w771 -> [_]
                tunnel: w772 -> [w784] mode=indexing
                tunnel: [w783] -> w767 mode=indexing
                tunnel: [w782] -> w768 mode=indexing
                tunnel: [w781] -> _
                i -> [w781]
                n573 = Unbundle(w784) -> (w783:dbl, w782:dbl)  [unwired: 1 out]
              }
              n574 = Build Array(w762, w761) -> (w763:dbl[][])
              n575 = Build Array(w767, w768) -> (w766:dbl[][])
              n576 = Transpose 2D Array(2D array=w763) -> (transposed array=→"lane_right_pt":dbl[][])
              n577 = Transpose 2D Array(2D array=w766) -> (transposed array=→"lane_left_pt":dbl[][])
            }
            frame #3 {
              n578 = local read "lane_right_pt"() -> (w811:dbl[][])
              n579 = local read "lane_left_pt"() -> (w809:dbl[][])
              n580 = Empty Array?(array=w811) -> (empty?=w810:bool)
              n581 = Empty Array?(array=w809) -> (empty?=w808:bool)
              n582 = case shown="False" w810 {
                tunnel: [w865 _] -> w805
                tunnel: [w864 _] -> w802
                frame False {
                  n583 = local read "map_track"() -> (w863:dbl[][])
                  n584 = local read "lane_right_pt"() -> (w867:dbl[][])
                  n585 = local read "map_track"() -> (w871:dbl[][])
                  n586 = Index Array(array=w863, index (col)=1 ("disabled index (col)")) -> ()  [unwired: 1 in, 1 out]
                  n587 = Index Array(array=w867, index (col) #1=0 ("disabled index (col)")) -> (element #1=w869:dbl[], element #2=w870:dbl[])  [unwired: 3 in]
                  n588 = Delete From Array(array=w871, index (row)=0) -> (deleted portion=w874:dbl[], array with subset deleted=w872:dbl[][])  [unwired: 2 in]
                  n589 = local read "d_safe"() -> (w866:dbl)
                  n590 = for {
                    tunnel: w869 -> [w906]
                    tunnel: w870 -> [w905]
                    tunnel: w872 -> [w896] mode=indexing
                    shift-right: [w896] -> _
                    shift-left: w874 -> [w895]
                    tunnel: [w884] -> w875 mode=indexing
                    tunnel: [w882] -> w876 mode=indexing
                    tunnel: w866 -> [w883]
                    n591 = Subtract(x=w896, y=w895) -> (x-y=w894:dbl[])
                    n592 = Index Array(array=w896) -> (element #1=w898:dbl, element #2=w897:dbl)  [unwired: 2 in]
                    n593 = Subtract(x=w906, y=w898) -> (x-y=w904:dbl[])
                    n594 = Subtract(x=w905, y=w897) -> (x-y=w903:dbl[])
                    n595 = Index Array(array=w894, index #1=1 ("index"), index #2=0 ("index")) -> (element #1=w891:dbl, element #2=w890:dbl)
                    n596 = Square(x=w904) -> (x^2=w901:dbl[])
                    n597 = Square(x=w903) -> (x^2=w902:dbl[])
                    n598 = Inverse Tangent (2 Input)(1:w890, 2:w891) -> (0:w889:dbl)
                    n599 = Add(x=w901, y=w902) -> (x+y=w900:dbl[])
                    n600 = call "headingoperater.vi"("h1"=1.5707963267948966, "h2"=w889) -> ("h2+h1"=w882:dbl)  [unwired: 8 in, 1 out]
                    n601 = Square Root(x=w900) -> (sqrt(x)=w899:dbl[])
                    n602 = Array Max & Min(array=w899) -> (min value=w887:dbl)  [unwired: 3 out]
                    n603 = Subtract(x=w883, y=w887) -> (x-y=w886:dbl)
                    n604 = Max & Min(x=w886, y=0.0) -> (max(x,y)=w884:dbl)  [unwired: 1 out]
                  }
                  n605 = Polar To Re/Im(2:w876, 3:w875) -> (0:w878:dbl[], 1:w877:dbl[])
                  n606 = Add Array Elements(numeric array=w877) -> (sum=w880:dbl)
                  n607 = Add Array Elements(numeric array=w878) -> (sum=w879:dbl)
                  n608 = Array Size(array=w878) -> (size(s)=w881:i32)
                  n609 = Divide(x=w880, y=w881) -> (x/y=w865:dbl)
                  n610 = Divide(x=w879, y=w881) -> (x/y=w864:dbl)
                }
                frame True {
                }
              }
              n611 = case shown="False" w808 {
                tunnel: [w820 _] -> w796
                tunnel: [w819 _] -> w799
                frame False {
                  n612 = local read "lane_left_pt"() -> (w836:dbl[][])
                  n613 = local read "map_track"() -> (w832:dbl[][])
                  n614 = Index Array(array=w836, index (col) #1=0 ("disabled index (col)")) -> (element #1=w834:dbl[], element #2=w833:dbl[])  [unwired: 3 in]
                  n615 = Delete From Array(array=w832, index (row)=0) -> (deleted portion=w829:dbl[], array with subset deleted=w831:dbl[][])  [unwired: 2 in]
                  n616 = local read "d_safe"() -> (w821:dbl)
                  n617 = for {
                    tunnel: w834 -> [w861]
                    tunnel: w833 -> [w860]
                    tunnel: w831 -> [w851] mode=indexing
                    shift-right: [w851] -> _
                    shift-left: w829 -> [w850]
                    tunnel: [w838] -> w828 mode=indexing
                    tunnel: [w839] -> w827 mode=indexing
                    tunnel: w821 -> [w837]
                    n618 = Subtract(x=w851, y=w850) -> (x-y=w849:dbl[])
                    n619 = Index Array(array=w851) -> (element #1=w853:dbl, element #2=w852:dbl)  [unwired: 2 in]
                    n620 = Subtract(x=w861, y=w853) -> (x-y=w859:dbl[])
                    n621 = Subtract(x=w860, y=w852) -> (x-y=w858:dbl[])
                    n622 = Index Array(array=w849, index #1=1 ("index"), index #2=0 ("index")) -> (element #1=w846:dbl, element #2=w845:dbl)
                    n623 = Square(x=w859) -> (x^2=w856:dbl[])
                    n624 = Square(x=w858) -> (x^2=w857:dbl[])
                    n625 = Inverse Tangent (2 Input)(1:w845, 2:w846) -> (0:w844:dbl)
                    n626 = Add(x=w856, y=w857) -> (x+y=w855:dbl[])
                    n627 = call "headingoperater.vi"("h1"=1.5707963267948966, "h2"=w844) -> ("h2-h1"=w839:dbl)  [unwired: 8 in, 1 out]
                    n628 = Square Root(x=w855) -> (sqrt(x)=w854:dbl[])
                    n629 = Array Max & Min(array=w854) -> (min value=w842:dbl)  [unwired: 3 out]
                    n630 = Subtract(x=w837, y=w842) -> (x-y=w841:dbl)
                    n631 = Max & Min(x=w841, y=0.0) -> (max(x,y)=w838:dbl)  [unwired: 1 out]
                  }
                  n632 = Polar To Re/Im(2:w827, 3:w828) -> (0:w825:dbl[], 1:w826:dbl[])
                  n633 = Add Array Elements(numeric array=w826) -> (sum=w823:dbl)
                  n634 = Add Array Elements(numeric array=w825) -> (sum=w824:dbl)
                  n635 = Array Size(array=w825) -> (size(s)=w822:i32)
                  n636 = Divide(x=w823, y=w822) -> (x/y=w820:dbl)
                  n637 = Divide(x=w824, y=w822) -> (x/y=w819:dbl)
                }
                frame True {
                }
              }
              n638 = Not A Number/Path/Refnum?(number/path/refnum=w805) -> (NaN/Path/Refnum?=w807:bool)
              n639 = Not A Number/Path/Refnum?(number/path/refnum=w802) -> (NaN/Path/Refnum?=w803:bool)
              n640 = Not A Number/Path/Refnum?(number/path/refnum=w796) -> (NaN/Path/Refnum?=w797:bool)
              n641 = Not A Number/Path/Refnum?(number/path/refnum=w799) -> (NaN/Path/Refnum?=w801:bool)
              n642 = local read "map_track"() -> (w818:dbl[][])
              n643 = Select(t=0.0, s=w807, f=w805) -> (s? t:f=w793:dbl)
              n644 = Select(t=0.0, s=w803, f=w802) -> (s? t:f=w790:dbl)
              n645 = Select(t=0.0, s=w797, f=w796) -> (s? t:f=w792:dbl)
              n646 = Select(t=0.0, s=w801, f=w799) -> (s? t:f=w791:dbl)
              n647 = Add(x=w793, y=w792) -> (x+y=w794:dbl)
              n648 = Add(x=w790, y=w791) -> (x+y=w788:dbl)
              n649 = Index Array(array=w818, index (col) #1=0 ("disabled index (col)")) -> (element #1=w816:dbl[], element #2=w815:dbl[])  [unwired: 3 in]
              n650 = Add(x=w794, y=w816) -> (x+y=w814:dbl[])
              n651 = Add(x=w788, y=w815) -> (x+y=w813:dbl[])
              n652 = Multiply(x="x_gain", y=w794) -> (x*y=w787:dbl)
              n653 = Multiply(x=w788, y="y_gain") -> (x*y=w786:dbl)
              n654 = Build Array(w814, w813) -> (w812:dbl[][])
              n655 = Transpose 2D Array(2D array=w812) -> (transposed array=w785:dbl[][])
            }
          }
        }
        frame True {
        }
      }
      "map_track 2" <- w663
      "y_shift" <- w666
      "x_shift" <- w665
      n656 = global write "G_SEN.vi" "vision x shift"(w665) -> ()
      n657 = global write "G_SEN.vi" "vision y shift"(w666) -> ()
    }
    frame #4 {
      n658 = disable-structure shown="Enabled" {
        frame Enabled {
          n659 = local read "w 2"() -> (w929:dbl[])
          n660 = local read "w 2"() -> (w928:dbl[])
          n661 = local read "w"() -> (→"Waveform Graph":dbl[])
          n662 = local read "w"() -> (w1016:dbl[])
          n663 = local read "w"() -> (w918:dbl[])
          n664 = local read "w"() -> (w998:dbl[])
          n665 = local read "w"() -> (w921:dbl[])
          n666 = Greater Or Equal?(x=w928, y=1.0) -> (x >= y?=w923:bool[])
          n667 = Less Or Equal?(x=w1016, y=-1.0) -> (x <= y?=w926:bool[])
          n668 = Less Or Equal?(x=w929, y=-1.0) -> (x <= y?=w924:bool[])
          n669 = Greater Or Equal?(x=w918, y=1.0) -> (x >= y?=w916:bool[])
          n670 = Greater Or Equal?(x=w998, y=1.0) -> (x >= y?=w925:bool[])
          n671 = Less Or Equal?(x=w921, y=-1.0) -> (x <= y?=w920:bool[])
          n672 = Or(x=w926, y=w924) -> (x .or. y?=w914:bool[])
          n673 = Or(x=w925, y=w923) -> (x .or. y?=w912:bool[])
          n674 = Not(x=w916) -> (.not. x?=w915:bool[])
          n675 = Not(x=w920) -> (.not. x?=w919:bool[])
          n676 = And(x=w914, y=w915) -> (x .and. y?=w913:bool[])
          n677 = And(x=w912, y=w919) -> (x .and. y?=w911:bool[])
          n678 = local read "x 2"() -> (w1014:dbl[])
          n679 = local read "y 2"() -> (w1013:dbl[])
          n680 = local read "x 2"() -> (w1000:dbl[])
          n681 = local read "y 2"() -> (w1001:dbl[])
          n682 = Build Cluster Array(w913, w1014, w1013) -> (w1012:cluster{bool, dbl, dbl}[])
          n683 = Build Cluster Array(w911, w1000, w1001) -> (w1002:cluster{bool, dbl, dbl}[])
          n684 = Sort 1D Array(array=w1012) -> (sorted array=w1011:cluster{bool, dbl, dbl}[])
          n685 = Sort 1D Array(array=w1002) -> (sorted array=w1003:cluster{bool, dbl, dbl}[])
          n686 = Reverse 1D Array(array=w1011) -> (reversed array=w1010:cluster{bool, dbl, dbl}[])
          n687 = Reverse 1D Array(array=w1003) -> (reversed array=w1004:cluster{bool, dbl, dbl}[])
          n688 = for {
            tunnel: w1010 -> [w1030] mode=indexing
            tunnel: [w1028] -> w1009 mode=indexing
            tunnel: [w1027] -> w993 mode=indexing
            tunnel: [w1026] -> w1008
            i -> [w1026]
            stop <- w1029 continue-if-true
            n689 = Unbundle(w1030) -> (w1029:bool, w1028:dbl, w1027:dbl)
          }
          n690 = for {
            tunnel: w1004 -> [w1025] mode=indexing
            tunnel: [w1023] -> w1005 mode=indexing
            tunnel: [w1022] -> w991 mode=indexing
            tunnel: [w1021] -> w1006
            i -> [w1021]
            stop <- w1024 continue-if-true
            n691 = Unbundle(w1025) -> (w1024:bool, w1023:dbl, w1022:dbl)
          }
          n692 = Array Subset(array=w1009, index=0, length=w1008) -> (w1007:dbl[])
          n693 = Array Subset(array=w1005, index=0, length=w1006) -> (w997:dbl[])
          n694 = Array Subset(array=w993, index=0, length=w1008) -> (w990:dbl[])
          n695 = Array Subset(array=w991, index=0, length=w1006) -> (w986:dbl[])
          n696 = call "Convert to Dynamic Data4"("Array"=w1007) -> ("Dynamic Data Type"=w975:dynamicdata)  [unwired: 3 in]
          n697 = Array Max & Min(array=w990) -> (max value=w910:dbl, min value=w909:dbl)  [unwired: 2 out]
          n698 = call "Convert to Dynamic Data3"("Array"=w990) -> ("Dynamic Data Type"=w987:dynamicdata)  [unwired: 3 in]
          n699 = call "Convert to Dynamic Data6"("Array"=w997) -> ("Dynamic Data Type"=w973:dynamicdata)  [unwired: 3 in]
          n700 = Array Max & Min(array=w986) -> (max value=w908:dbl, min value=w907:dbl)  [unwired: 2 out]
          n701 = call "Convert to Dynamic Data8"("Array"=w986) -> ("Dynamic Data Type"=w985:dynamicdata)  [unwired: 3 in]
          n702 = local read "map_track"() -> (w939:dbl[][])
          n703 = Add(x=w910, y=w908) -> (x+y=w958:dbl)
          n704 = Add(x=w909, y=w907) -> (x+y=w954:dbl)
          n705 = call-poly <vilib>:"Ramp Pattern.vi"("start"=w909, "end"=w910, "delta"=0.01) -> ("Ramp Pattern"=w962:dbl[])  [unwired: 6 in, 2 out]
          n706 = call-poly <vilib>:"Ramp Pattern.vi"("start"=w907, "end"=w908, "delta"=0.01) -> ("Ramp Pattern"=w961:dbl[])  [unwired: 6 in, 2 out]
          n707 = local read "Coeff right"() -> (w960:dbl[])
          n708 = local read "Coeff stop"() -> (w996:dbl[])
          n709 = local read "Coeff left"() -> (w1019:dbl[])
          n710 = Index Array(array=w939, index (col) #1=0 ("disabled index (col)")) -> (element #1=w941:dbl[], element #2=w943:dbl[])  [unwired: 3 in]
          n711 = Multiply(x=w958, y=0.5) -> (x*y=w956:dbl)
          n712 = Multiply(x=w954, y=0.5) -> (x*y=w953:dbl)
          n713 = local read "map_track 2"() -> (w938:dbl[][])
          n714 = call-poly <vilib>:"Polynomial Evaluation.vi"("P(x)"=w1019, "A"=w962) -> ("P(A)"=w968:dbl[])  [unwired: 1 out]
          n715 = call-poly <vilib>:"Polynomial Evaluation.vi"("P(x)"=w960, "A"=w961) -> ("P(A)"=w963:dbl[])  [unwired: 1 out]
          n716 = local read "y_shift"() -> (w931:dbl)
          n717 = call "Convert to Dynamic Data7"("Array"=w962) -> ("Dynamic Data Type"=w972:dynamicdata)  [unwired: 3 in]
          n718 = call "Convert to Dynamic Data11"("Array"=w961) -> ("Dynamic Data Type"=w971:dynamicdata)  [unwired: 3 in]
          n719 = local read "x_shift"() -> (w932:dbl)
          n720 = local read "y_end"() -> (w995:dbl[])
          n721 = call-poly <vilib>:"Ramp Pattern.vi"("start"=w953, "end"=w956, "delta"=0.01) -> ("Ramp Pattern"=w949:dbl[])  [unwired: 6 in, 2 out]
          n722 = global read "G_SEN.vi" "Lane_C_M"() -> (w952:dbl[])
          n723 = Add(x=w941, y=w932) -> (x+y=w940:dbl[])
          n724 = Add(x=w943, y=w931) -> (x+y=w942:dbl[])
          n725 = call-poly <vilib>:"Polynomial Evaluation.vi"("P(x)"=w996, "A"=w995) -> ("P(A)"=w969:dbl[])  [unwired: 1 out]
          n726 = Build Array(w968, w962) -> (w967:dbl[][])
          n727 = Build Array(w963, w961) -> (w964:dbl[][])
          n728 = call "Convert to Dynamic Data2"("Array"=w968) -> ("Dynamic Data Type"=w976:dynamicdata)  [unwired: 3 in]
          n729 = call "Convert to Dynamic Data5"("Array"=w963) -> ("Dynamic Data Type"=w974:dynamicdata)  [unwired: 3 in]
          n730 = Index Array(array=w938, index (col) #1=0 ("disabled index (col)")) -> (element #1=w936:dbl[], element #2=w934:dbl[])  [unwired: 3 in]
          n731 = local read "y 2"() -> (w1018:dbl[])
          n732 = local read "y_end"() -> (w970:dbl[])
          n733 = call-poly <vilib>:"Polynomial Evaluation.vi"("P(x)"=w952, "A"=w949) -> ("P(A)"=w951:dbl[])  [unwired: 1 out]
          n734 = Transpose 2D Array(2D array=w967) -> (transposed array=w966:dbl[][])
          n735 = Transpose 2D Array(2D array=w964) -> (transposed array=w965:dbl[][])
          n736 = call "Convert to Dynamic Data14"("Array"=w949) -> ("Dynamic Data Type"=w948:dynamicdata)  [unwired: 3 in]
          n737 = call "Convert to Dynamic Data15"("Array"=w940) -> ("Dynamic Data Type"=w946:dynamicdata)  [unwired: 3 in]
          n738 = call "Convert to Dynamic Data16"("Array"=w942) -> ("Dynamic Data Type"=w945:dynamicdata)  [unwired: 3 in]
          n739 = call "Convert to Dynamic Data17"("Array"=w936) -> ("Dynamic Data Type"=w935:dynamicdata)  [unwired: 3 in]
          n740 = call "Convert to Dynamic Data18"("Array"=w934) -> ("Dynamic Data Type"=w933:dynamicdata)  [unwired: 3 in]
          n741 = call "Convert to Dynamic Data"("Array"=w969) -> ("Dynamic Data Type"=w981:dynamicdata)  [unwired: 3 in]
          n742 = call "Convert to Dynamic Data10"("Array"=w1018) -> ("Dynamic Data Type"=w983:dynamicdata)  [unwired: 3 in]
          n743 = local read "x 2"() -> (w1017:dbl[])
          n744 = global write "G_SEN.vi" "Lane_L_V"(w966) -> ()
          n745 = global write "G_SEN.vi" "Lane_R_V"(w965) -> ()
          n746 = Merge Signals(w972, w987, w971, w985, w983, w981, w948, w945, w933) -> (w988:dynamicdata)
          n747 = call "Convert to Dynamic Data12"("Array"=w970) -> ("Dynamic Data Type"=w982:dynamicdata)  [unwired: 3 in]
          n748 = call "Convert to Dynamic Data13"("Array"=w951) -> ("Dynamic Data Type"=w950:dynamicdata)  [unwired: 3 in]
          n749 = call "Convert to Dynamic Data9"("Array"=w1017) -> ("Dynamic Data Type"=w984:dynamicdata)  [unwired: 3 in]
          n750 = Merge Signals(w976, w975, w974, w973, w984, w982, w950, w946, w935) -> (w989:dynamicdata)
          n751 = call "Build XY Graph"("Y Input"=w988, "X Input"=w989) -> ("XY Graph"=→"XY Graph 4":cluster{"X":dbl[], "Y":dbl[]}[])  [unwired: 8 in, 1 out]
        }
        frame Disabled {
        }
      }
    }
  }
